vi "Create Message Getter (from Accessor).vi"(8 "error in (no error)":errorcluster, 10 "RPC Message Name":string, 11 "RPC Messages Folder (ProjectItem) in":refnum<vi>) -> (0 "error out":errorcluster, 1 "Created ?":bool, 2 "Getter VI out":refnum<vi>, 3 "RPC Messages Folder (ProjectItem) out":refnum<vi>)   [LabVIEW 2022 SP3, in "gRPC Template Creation Utility.lvlib"]
uses:
  gRPC Template Creation Utility.lvlib
  <vilib>/Utility/error.llb/Trim Whitespace One-Sided.vi
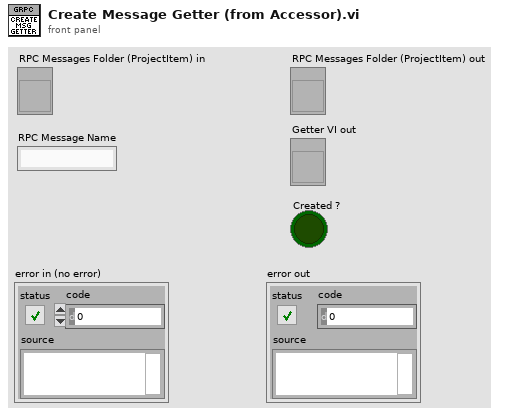
[diagram p1: front panel]
types:
  T1 = enum32{"invalid VI type", "Standard VI", "Control VI", "Global VI", "Polymorphic VI", "Configuration VI", "SubSystem", "Facade VI", "Method VI"}
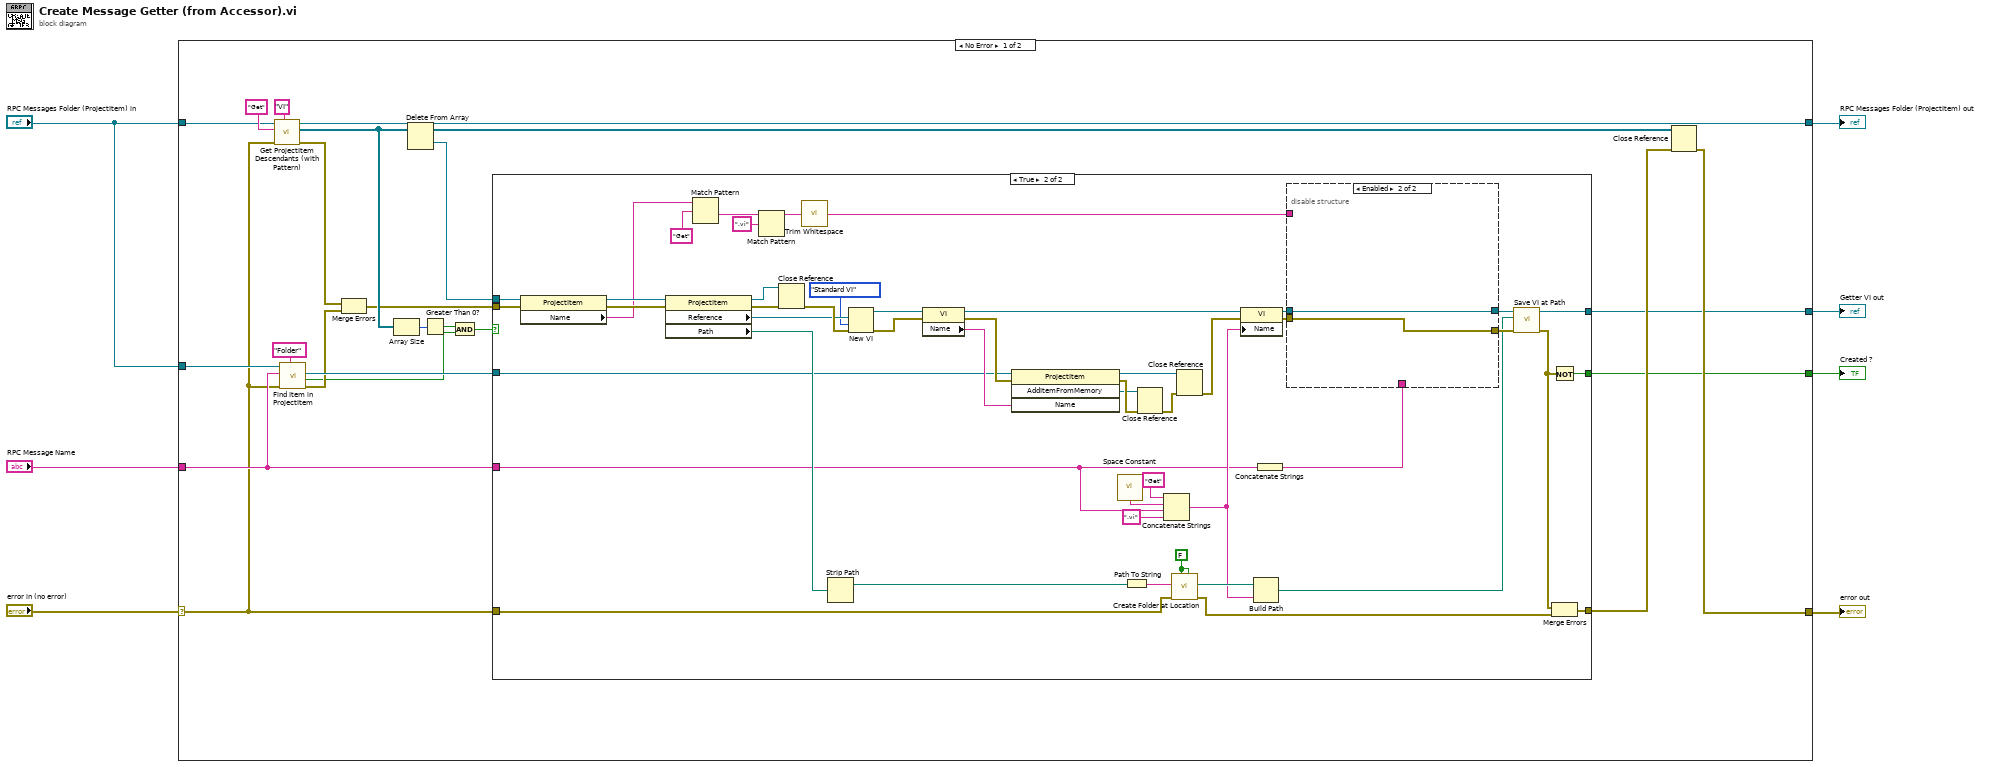
[diagram p0: block diagram]
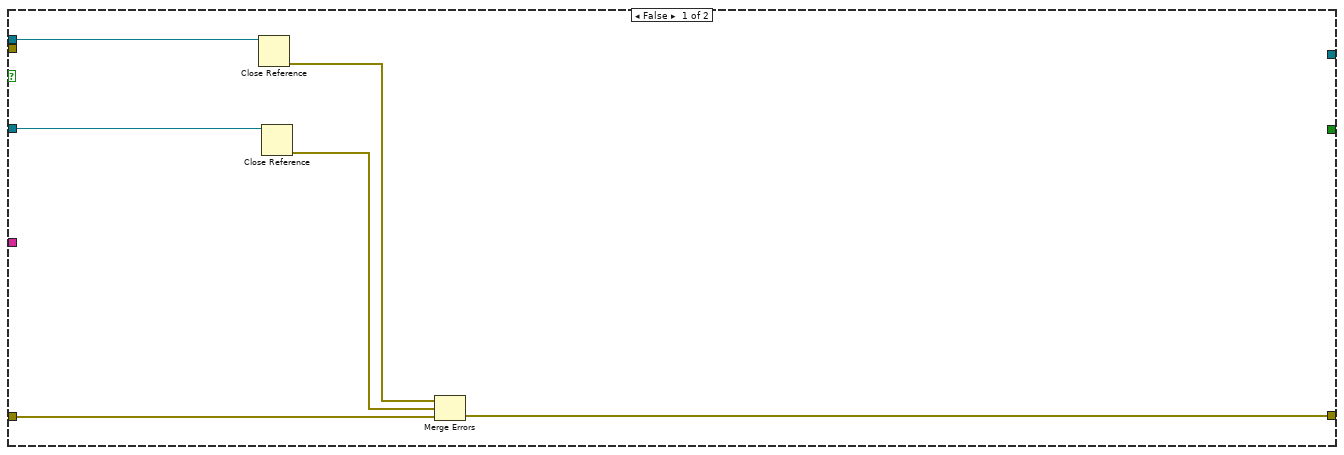
[diagram p2: hidden frame]
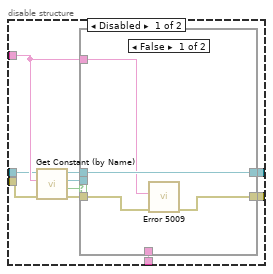
[diagram p3: hidden frame]
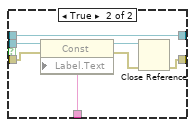
[diagram p4: hidden frame]
diagram:
  n1 = case shown="No Error" "error in (no error)" {
    selector: "error in (no error)" -> [w13 w109]
    tunnel: "RPC Message Name" -> [w25 _]
    tunnel: "RPC Messages Folder (ProjectItem) in" -> [w23 _]
    tunnel: "RPC Messages Folder (ProjectItem) in" -> [w18 w108]
    tunnel: [w11 w109] -> w4
    tunnel: [w10 w108] -> w3
    tunnel: [w9 _] -> w2
    tunnel: [w8 _] -> w1
    frame No Error {
      n2 = call "Get ProjectItem Descendants (with Pattern).vi"("Type"="VI", "error in (no error)"=w13, "Pattern"="Get", "ProjectItem in"=w18) -> ("error out"=w17:errorcluster, "ProjectItem descendents"=w24:refnum<vi>[], "ProjectItem out"=w10:refnum<vi>)  [unwired: 5 in]
      n3 = call "Find Item in ProjectItem.vi"("Item Type"="Folder", "error in (no error)"=w13, "Name"=w25, "ProjectItem in"=w23) -> ("error out"=w16:errorcluster, "Found ?"=w15:bool, "Item Refnum out"=w21:refnum<vi>)  [unwired: 4 in, 1 out]
      n4 = Merge Errors(w17, w16) -> (w14:errorcluster)
      n5 = Array Size(array=w24) -> (size(s)=w22:i32)
      n6 = Delete From Array(array=w24) -> (deleted portion=w27:refnum<vi>, array with subset deleted=w30:refnum<vi>[])  [unwired: 2 in]
      n7 = Greater Than 0?(x=w22) -> (x > 0?=w20:bool)
      n8 = And(x=w20, y=w15) -> (x .and. y?=w19:bool)
      n9 = case shown="True" w19 {
        tunnel: w25 -> [_ w45]
        tunnel: [w33 w81] -> w12
        tunnel: [_ w42] -> w8
        tunnel: w27 -> [w36 w56]
        tunnel: [_ w66] -> w9
        tunnel: w21 -> [w31 w61]
        tunnel: w13 -> [w32 w60]
        tunnel: w14 -> [_ w55]
        frame False {
          n10 = Close Reference(reference=w36) -> (error out=w34:errorcluster)  [unwired: 1 in]
          n11 = Close Reference(reference=w31) -> (error out=w35:errorcluster)  [unwired: 1 in]
          n12 = Merge Errors(w34, w35, w32) -> (w33:errorcluster)
        }
        frame True {
          w79 = FALSE ("Use Relative (F)")
          n13 = property class="ProjectItem"(reference=w56, error in=w55) -> (reference out=w54:refnum<vi>, error out=w53:errorcluster, "Name"=w52:string)
          n14 = property class="ProjectItem"(reference=w54, error in=w53) -> (reference out=w84:refnum<vi>, error out=w82:errorcluster, "Reference"=w72:refnum<vi>, "Path"=w75:path)
          n15 = Match Pattern(string=w52, regular expression="Get") -> (after substring=w50:string)  [unwired: 1 in, 3 out]
          n16 = Match Pattern(string=w50, regular expression=".vi") -> (before substring=w39:string)  [unwired: 1 in, 3 out]
          n17 = Close Reference(reference=w84, error in (no error)=w82) -> (error out=w83:errorcluster)
          n18 = call <vilib>:"Trim Whitespace.vi"("string"=w39) -> ("trimmed string"=w48:string)  [unwired: 1 in]
          n19 = Strip Path(path=w75) -> (stripped path=w37:path)  [unwired: 1 out]
          n20 = New VI(8:w83, 9:T1."Standard VI" ("vi type (standard vi)"), 10:w72) -> (0:w71:errorcluster, 3:w69:refnum<vi>)  [unwired: 1 in, 3 out]
          n21 = property class="VI"(reference=w69, error in=w71) -> (reference out=w76:refnum<vi>, error out=w77:errorcluster, "Name"=w73:string)
          n22 = invoke class="ProjectItem" method="AddItemFromMemory"(reference=w61, error in=w77, "Name"=w73) -> (reference out=w68:refnum<vi>, error out=w59:errorcluster, "AddItemFromMemory"=w58:refnum<vi>)  [unwired: 1 in, 1 out]
          n23 = call <vilib>:"Space Constant.vi"() -> ("String"=w64:string)
          n24 = Path To String(path=w37) -> (string=w74:string)
          n25 = Close Reference(reference=w58, error in (no error)=w59) -> (error out=w57:errorcluster)
          n26 = Concatenate Strings("Get" ("string"), w64, w45, ".vi" ("string")) -> (w62:string)
          n27 = call "Create Folder at Location.vi"("Override existing (F)"=w79, "Use Relative (F)"=w79, "Error In"=w60, "Path"=w74) -> ("Error Out"=w80:errorcluster, "Full path out"=w78:path)  [unwired: 5 in, 1 out]
          n28 = Close Reference(reference=w68, error in (no error)=w57) -> (error out=w67:errorcluster)
          n29 = property class="VI"(reference=w76, error in=w67, "Name"=w62) -> (reference out=w47:refnum<vi>, error out=w46:errorcluster)
          n30 = Build Path(base path=w78, name or relative path=w62) -> (appended path=w41:path)
          n31 = Concatenate Strings(w45) -> (w44:string)
          n32 = disable-structure shown="Enabled" {
            disable-tunnel: w48 -> [w94 _]
            disable-tunnel: w47 -> [w92 w107]
            disable-tunnel: w46 -> [w91 w106]
            disable-tunnel: w44 -> [w90 _]
            disable-tunnel: [w88 w106] -> w43
            disable-tunnel: [w85 w107] -> w38
            frame Disabled {
              n33 = call "Get Constant (by Name).vi"("error in (no error)"=w91, "Constant Label"=w94, "Owner VI in"=w92) -> ("error out"=w89:errorcluster, "Found ?"=w87:bool, "Const ref out"=w93:refnum<vi>, "Owner VI out"=w86:refnum<vi>)  [unwired: 5 in]
              n34 = case shown="False" w87 {
                tunnel: w93 -> [_ w105]
                tunnel: w90 -> [_ w104]
                tunnel: w89 -> [w97 w103]
                tunnel: [w96 w100] -> w88
                tunnel: w86 -> [w98 w99]
                tunnel: [w98 w99] -> w85
                tunnel: w94 -> [w95 _]
                frame False {
                  n35 = call "Error 5009.vi"("error in (no error)"=w97, "Cluster Definition Constant"=w95) -> ("error out"=w96:errorcluster)  [unwired: 9 in]
                }
                frame True {
                  n36 = property class="Const"(reference=w105, error in=w103, "Label.Text"=w104) -> (reference out=w102:refnum<vi>, error out=w101:errorcluster)
                  n37 = Close Reference(reference=w102, error in (no error)=w101) -> (error out=w100:errorcluster)
                }
              }
            }
            frame Enabled {
            }
          }
          n38 = call "Save VI at Path.vi"("error in (no error)"=w43, "Path"=w41, "VI in"=w38) -> ("error out"=w40:errorcluster, "VI out"=w42:refnum<vi>)  [unwired: 6 in, 1 out]
          n39 = Not(x=w40) -> (.not. x?=w66:bool)
          n40 = Merge Errors(w40, w80) -> (w81:errorcluster)
        }
      }
      n41 = Close Reference(reference=w30, error in (no error)=w12) -> (error out=w11:errorcluster)
    }
    frame Error {
    }
  }
  "error out" <- w4
  "RPC Messages Folder (ProjectItem) out" <- w3
  "Created ?" <- w2
  "Getter VI out" <- w1
